vi "2-1.vi"() -> ()   [LabVIEW 2019, in "AoC2022.lvlib"]
uses:
  AoC2022.lvlib
panel:
  out "Player 1":i32
  out "Player 2":i32
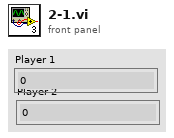
[diagram p1: front panel]
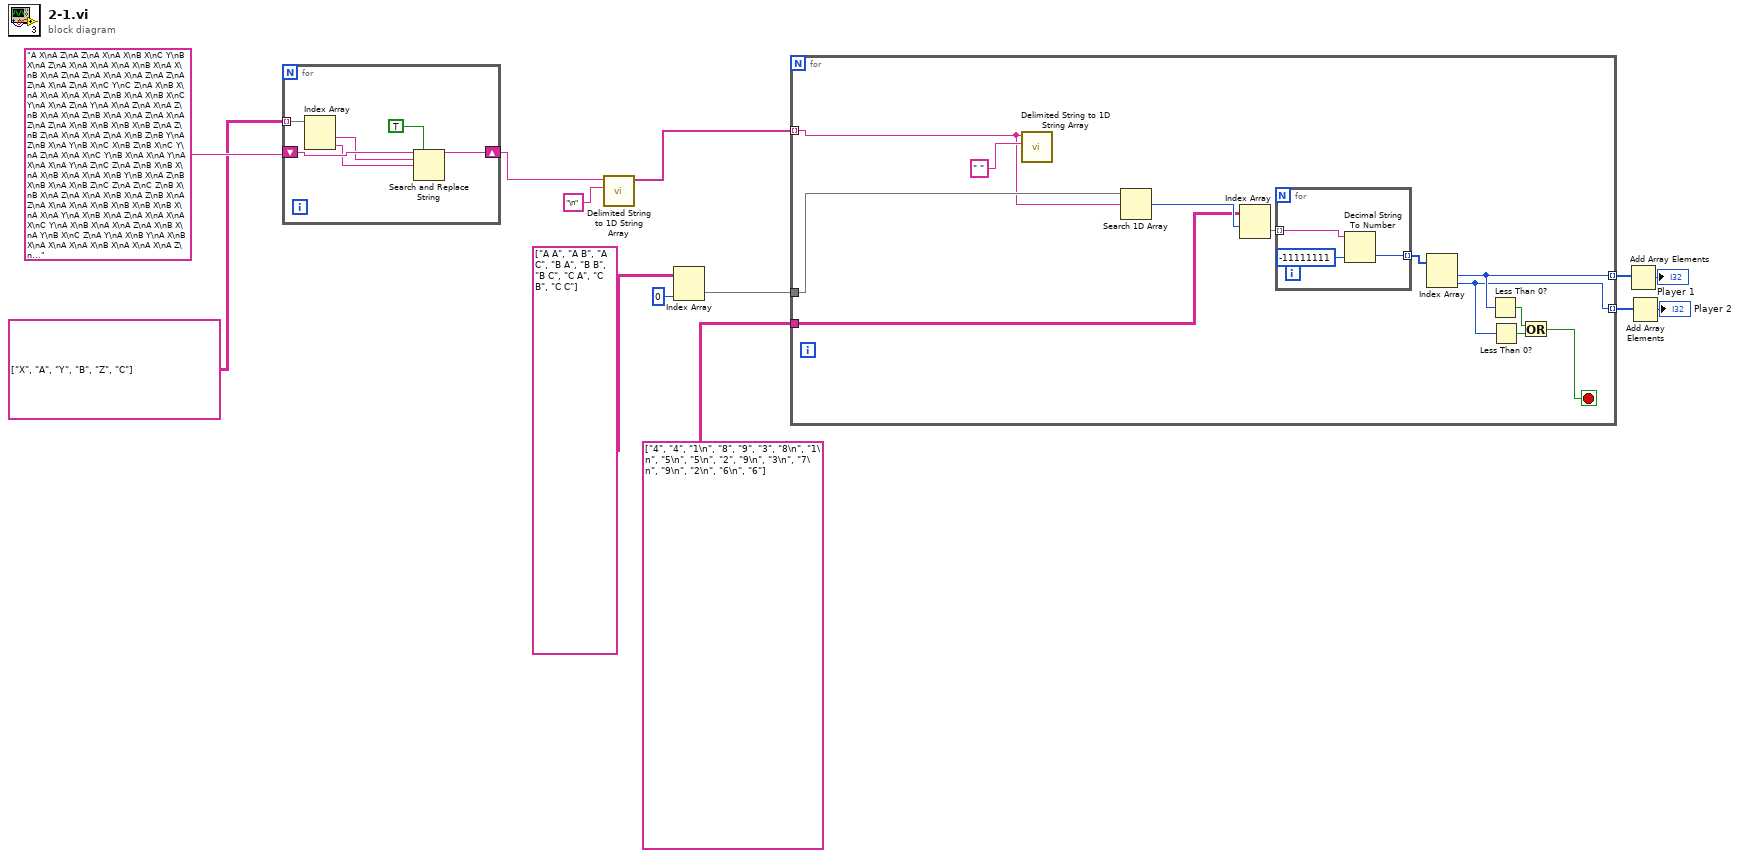
[diagram p0: block diagram]
diagram:
  n1 = for {
    tunnel: string[][] [["X", "A"], ["Y", "B"], ["Z", "C"]] -> [w18] mode=indexing
    shift-right: [w14] -> w1
    shift-left: "A X\nA Z\nA Z\nA X\nA X\nB X\nC Y\nB X\nA Z\nA X\nA X\nA X\nA X\nB X\nA X\nB X\nA Z\nA Z\nA X\nA X\nA Z\nA Z\nA Z\nA X\nA Z\nA X\nC Y\nC Z\nA X\nB X\nA X\nA X\nA X\nA Z\nB X\nA X\nB X\nC Y\nA X\nA Z\nA Y\nA X\nA Z\nA X\nA Z\nB X\nA X\nA Z\nB X\nA X\nA Z\nA X\nA Z\nA Z\nA X\nB X\nB X\nB X\nB Z\nA Z\nB Z\nA X\nA X\nA Z\nA X\nB Z\nB Y\nA Z\nB X\nA Y\nB X\nC X\nB Z\nB X\nC Y\nA Z\nA X\nA X\nC Y\nB X\nA X\nA Y\nA X\nA X\nA Y\nA Z\nC Z\nA Z\nB X\nB X\nA X\nB X\nA X\nA X\nB Y\nB X\nA Z\nB X\nB X\nA X\nB Z\nC Z\nA Z\nC Z\nB X\nB X\nA Z\nA X\nA X\nB X\nA Z\nB X\nA Z\nA X\nA X\nA X\nB X\nB X\nB X\nB X\nA X\nA Y\nA X\nB X\nA Z\nA X\nA X\nA X\nC Y\nA X\nB X\nA X\nA Z\nA X\nB X\nA Y\nB X\nC Z\nA Y\nA X\nB Y\nA X\nB X\nA X\nA X\nA X\nB X\nA X\nA X\nA Z\nA Z\nA X\nC Y\nB X\nB X\nA Z\nB X\nB Y\nC Y\nA X\nA X\nB Y\nA X\nB Y\nB X\nB X\nA X\nA Z\nB X\nB X\nA Y\nA X\nC Y\nC Y\nC Y\nA X\nB X\nA X\nA X\nA X\nB X\nB X\nC Y\nA X\nA Z\nA Z\nA X\nB X\nA Z\nA Z\nA X\nB X\nA X\nA Z\nA X\nC Z\nB X\nA X\nC Y\nC Y\nA Z\nB X\nB Z\nC Y\nB X\nA Y\nB Y\nA Z\nA X\nA X\nB X\nB Y\nA Z\nA X\nB X\nA X\nC X\nC Y\nA X\nB X\nA Z\nA X\nB X\nA X\nC Y\nC Y\nC Y\nA X\nA X\nA Z\nA X\nC Y\nA Z\nB Y\nA X\nC Y\nB Z\nB X\nB X\nA Z\nB X\nA Y\nC X\nA X\nB X\nA Z\nC Y\nA X\nA Z\nC Z\nA X\nC Y\nB X\nC Y\nC Z\nA Y\nA Z\nC Y\nA X\nA X\nA X\nA Y\nB X\nB X\nC Y\nC Y\nA X\nA Z\nC Y\nB Z\nB X\nC Z\nB X\nB X\nC Z\nA X\nA X\nB X\nB X\nA X\nA X\nB X\nB X\nB X\nC Y\nA X\nA X\nA X\nA X\nB X\nA X\nA X\nB X\nB Z\nA X\nB X\nA X\nC Y\nB Y\nA X\nB X\nA Y\nB Z\nB X\nA X\nB Z\nB X\nA Y\nA X\nB X\nA X\nA Z\nB X\nA X\nA X\nC Z\nA X\nB X\nA X\nB Y\nA Z\nA X\nB X\nA X\nA Z\nB X\nB X\nB Y\nB X\nA X\nC Y\nA X\nA X\nB X\nB Y\nA X\nA X\nA X\nC Z\nC Z\nB Y\nB X\nB Z\nA X\nA Y\nA X\nC Y\nB X\nA X\nA X\nA X\nA Z\nC Y\nA X\nA X\nC Y\nA X\nA X\nA X\nA Z\nA Y\nA X\nA Y\nC Z\nA Z\nA X\nB X\nA Z\nC Z\nC Y\nA Z\nA Z\nC Y\nC Z\nC Z\nA X\nB X\nB X\nB Z\nC Y\nA X\nA X\nA X\nA Z\nA X\nB X\nB X\nC X\nA X\nA X\nB X\nA Y\nA X\nA X\nB Y\nC Z\nA X\nA X\nA Y\nB X\nB X\nB X\nC Z\nA Z\nA Y\nB Y\nA X\nB X\nB X\nB X\nB Z\nA Y\nB Y\nA Z\nA Z\nC Z\nB X\nA X\nA Y\nA Y\nC Y\nB Y\nA X\nA X\nA X\nA X\nB Y\nA X\nA Y\nA X\nA Z\nB X\nB X\nA Y\nA X\nA Y\nA Y\nA Z\nB X\nB X\nA Z\nB X\nA X\nA Z\nA Z\nB X\nA Z\nA X\nA Y\nA Z\nA X\nA Z\nB Y\nA X\nC Y\nB X\nC X\nC Y\nB Z\nC Y\nC Y\nA X\nA X\nA Y\nB X\nC Z\nB X\nC Y\nA X\nA Z\nC Y\nA X\nA Z\nA Z\nB Y\nA X\nA X\nB X\nB Y\nA X\nA X\nB X\nA X\nB X\nA X\nB X\nA X\nB Y\nA Z\nB X\nB X\nB X\nB X\nA Y\nA X\nA Y\nA Y\nC Z\nB Z\nA X\nB Y\nA X\nC Z\nB X\nA X\nA X\nA X\nA X\nA X\nC Z\nC Z\nC Z\nA X\nC Y\nA X\nC X\nC Z\nA X\nB X\nA Z\nA Z\nA Z\nA X\nA Z\nA Z\nB Z\nA X\nB X\nA Z\nC Y\nA X\nA Z\nA Z\nA Z\nB Z\nB X\nA X\nB X\nB X\nB X\nB X\nB Y\nB X\nA X\nA X\nA Z\nA Z\nA Z\nB Y\nA X\nA X\nA Y\nB X\nB X\nA Z\nA X\nB X\nA X\nA X\nA Z\nC Y\nA X\nB X\nA X\nB X\nA X\nB X\nA Z\nB X\nA X\nA Z\nA Z\nB X\nA Y\nA X\nA Z\nC Y\nA X\nA X\nA X\nB Y\nB X\nA Y\nA Z\nC X\nB X\nC Y\nA X\nB X\nC Z\nC Z\nA X\nB X\nB X\nB Y\nB X\nB X\nA X\nA Z\nB Z\nB X\nA X\nB X\nB X\nB X\nA Z\nA X\nA X\nA Z\nB Y\nB Z\nA X\nA Z\nA Z\nA Z\nA X\nA X\nA X\nA X\nA X\nA X\nB X\nA Z\nB Z\nA X\nA Z\nC Y\nA Z\nA X\nA Y\nA Y\nB X\nB Y\nA Z\nA X\nB X\nB Y\nA X\nB X\nA X\nB X\nB X\nC Y\nA Z\nB X\nA X\nB X\nA X\nA Z\nA X\nA Z\nA X\nA X\nA X\nB X\nA Y\nA X\nA X\nB X\nC Z\nB X\nA X\nC Y\nA X\nB X\nA Z\nB Y\nB Z\nA X\nA X\nA X\nC Y\nA X\nA X\nA X\nB X\nC Z\nA Z\nA X\nC Z\nB X\nA Z\nA Y\nC Y\nC Y\nA Z\nB X\nC Z\nC Z\nA X\nA X\nA X\nA X\nA X\nB X\nC Y\nA Z\nA X\nB X\nA Z\nA X\nA Y\nA X\nB Z\nA X\nB X\nA X\nA X\nA X\nA Y\nB X\nC Y\nA X\nA Z\nC Y\nA Z\nA X\nA Y\nA X\nA Z\nA X\nA Y\nC Y\nA Y\nA Z\nA X\nA X\nA X\nA Z\nA X\nB X\nA Y\nA X\nB X\nA X\nA X\nB X\nA X\nB X\nC Z\nB X\nA Z\nA Z\nC Y\nB Y\nB X\nA Y\nB X\nB X\nA Y\nA X\nC X\nC Y\nB X\nA X\nC X\nC Z\nA X\nA Z\nB X\nB Z\nC Y\nA X\nC Y\nA Y\nB X\nB Y\nA X\nC Y\nA Z\nA X\nA X\nC Y\nC Y\nA X\nA Z\nB X\nA Y\nB X\nA Z\nA Z\nA Z\nA Z\nA X\nC Z\nB X\nB Y\nA X\nA Y\nA X\nB X\nC Y\nC Z\nB Z\nB X\nB Z\nA X\nA Z\nC Y\nA X\nB Y\nA X\nA Z\nA X\nC Z\nA X\nA Y\nB Y\nA X\nA X\nA X\nA Z\nB X\nB X\nB X\nA X\nC Y\nC X\nC Y\nC Z\nA X\nA X\nA Z\nA Z\nA X\nA X\nA X\nA X\nA X\nA X\nA X\nC Z\nA X\nB X\nA Z\nB X\nB X\nB X\nA Y\nA X\nA X\nB X\nA X\nB X\nA Z\nC Y\nB Y\nC Z\nB Y\nB X\nB X\nA X\nC Z\nA X\nB Y\nC Y\nB Y\nA Z\nA Y\nA X\nA X\nC Y\nB X\nB X\nA Z\nA X\nC Y\nC Y\nA Y\nA Z\nB X\nC Z\nA Z\nC Y\nA X\nA X\nA Z\nB X\nA X\nA X\nA Z\nB X\nC Z\nA X\nA X\nB X\nB Y\nA Z\nA X\nB X\nA X\nC Y\nB X\nB X\nB Z\nC Y\nA X\nB X\nA X\nA X\nA Y\nA Y\nA Z\nB X\nA Z\nB Y\nB X\nA X\nB Y\nA X\nA X\nA Z\nA X\nB X\nA Z\nA X\nA Z\nB X\nB X\nB X\nB Z\nC Y\nA Y\nA Y\nA Z\nA X\nB X\nB X\nA X\nA X\nB Y\nA X\nB X\nA Z\nB Z\nB X\nC Y\nA Z\nA X\nC Z\nA Y\nA Y\nB X\nA Y\nC Z\nA Z\nA X\nB X\nA Z\nC Y\nC X\nB X\nB Z\nA X\nA Y\nA X\nB X\nA X\nA X\nC Y\nB Z\nB Z\nB Y\nC Z\nC Y\nB X\nB Y\nC Y\nA Z\nB X\nA X\nA X\nA X\nA X\nA X\nA X\nB X\nB X\nB X\nA X\nC Y\nA X\nA Y\nA Z\nB Y\nC Y\nA Z\nA X\nA X\nA Z\nA Y\nB X\nA Y\nA X\nA X\nC Z\nA X\nA X\nB X\nA X\nA Z\nA Z\nA X\nA X\nA X\nB X\nA X\nA X\nA X\nA Z\nA X\nB X\nB Z\nC Y\nA X\nA Z\nB X\nB X\nB X\nA X\nB X\nA X\nB X\nA Y\nB Y\nC Y\nA X\nC Z\nB Z\nA Z\nA X\nA X\nA Z\nA Y\nA Z\nA X\nA X\nB X\nA X\nA X\nA Z\nC Z\nB X\nB Y\nA Z\nB X\nA Z\nA X\nA X\nA X\nC Y\nC Y\nA Z\nA X\nA X\nB Y\nA Y\nA X\nB Z\nB X\nB Z\nB X\nB Y\nB X\nA Y\nA Z\nC Y\nB X\nA X\nA X\nB X\nB Z\nA X\nC X\nA X\nA X\nA X\nA X\nA X\nA X\nB X\nA X\nC Z\nA Y\nB X\nB X\nB Z\nA X\nB X\nB Z\nB X\nA Z\nA X\nB X\nA X\nA Y\nB X\nA Z\nC Z\nB X\nC Z\nA X\nA X\nC Y\nA Z\nC Y\nA Z\nA X\nB X\nA X\nC Y\nA Z\nA X\nA X\nB X\nB X\nA Z\nB Y\nB X\nA X\nA Z\nA X\nB X\nA X\nA Z\nA Z\nA Y\nA Y\nA X\nC Z\nA Z\nA Z\nA X\nB X\nA Y\nB Z\nA X\nA Z\nA X\nC Z\nB X\nA Z\nC Z\nA X\nC X\nA Z\nA X\nA X\nB Z\nA X\nB X\nA X\nB X\nC Z\nA X\nB X\nA Z\nB X\nC Y\nB X\nA Z\nA X\nA Y\nC Z\nA Z\nB X\nA Z\nA Y\nA Z\nB X\nA X\nB X\nC Y\nB X\nA X\nC Y\nA X\nA X\nB Y\nA X\nB Y\nA X\nA X\nA X\nB X\nA X\nA X\nC Z\nA X\nB X\nA Y\nA Y\nB Z\nA Z\nA Y\nA X\nB X\nB Y\nA Z\nB Y\nA X\nA Z\nA X\nA Z\nB X\nA X\nA X\nB X\nA Y\nB X\nB X\nA X\nA Z\nB X\nA Y\nB X\nA Z\nB X\nB X\nB X\nB X\nA Y\nA Z\nB X\nB Y\nB X\nC Y\nC Y\nC Y\nB X\nB X\nA Y\nA X\nB X\nB X\nA X\nB X\nA X\nA Z\nA Z\nA Z\nB X\nA X\nA X\nA Y\nA X\nA X\nC Y\nB X\nC Y\nA X\nA Y\nC Z\nA X\nB X\nA Z\nA X\nA X\nA Z\nA X\nB Z\nA X\nA Z\nA X\nC Y\nA Y\nC X\nA X\nC Y\nB X\nB X\nA Z\nA X\nA X\nA X\nB X\nA X\nC Y\nC Y\nA Y\nA X\nC Z\nA X\nB X\nB Y\nA Z\nA X\nB X\nB X\nA X\nA Z\nC Y\nB X\nA Y\nA X\nA Z\nB X\nA X\nA Z\nB X\nA Y\nB Z\nA Z\nC Z\nC Y\nA Z\nA X\nA X\nA Z\nB X\nA X\nB X\nA X\nA X\nB X\nA Z\nA X\nC Z\nB X\nA Z\nB Y\nA Z\nA X\nA Z\nB X\nA X\nA X\nA Y\nB X\nC Z\nB X\nA X\nA X\nA Z\nB X\nC X\nB X\nB X\nA Z\nB Y\nB X\nA Z\nC Y\nA X\nA X\nB X\nB X\nA X\nB X\nA Z\nA X\nA X\nA Z\nA X\nA X\nB X\nB X\nA X\nA Z\nA Y\nA X\nA X\nC Y\nB X\nA X\nB X\nC Z\nA Z\nB X\nA X\nA X\nA X\nC Y\nA X\nA X\nA X\nA Z\nB Y\nB X\nA X\nA X\nA Z\nB X\nC Z\nB X\nA Z\nA Z\nA X\nA Y\nB Y\nB X\nA Z\nA Z\nA X\nA Y\nB X\nA X\nA Z\nB X\nA Y\nA Z\nA Z\nB X\nC Z\nA X\nA X\nB X\nB X\nA X\nA Y\nA Y\nC Z\nB X\nA X\nA Z\nC Y\nB X\nA Z\nA X\nB X\nB Y\nA X\nB X\nA Y\nB X\nA X\nA Z\nB X\nB X\nC Y\nB X\nB X\nB Y\nA X\nA X\nB X\nB X\nA X\nB X\nC Y\nA X\nA X\nA Z\nA Z\nB X\nA Y\nB X\nB Y\nA X\nA Z\nA X\nA Z\nA X\nB Y\nB X\nB X\nA X\nB X\nA X\nB X\nB X\nA X\nB X\nC X\nA Z\nA Z\nA X\nA X\nA Z\nA X\nB X\nA X\nA X\nA Z\nA Z\nA X\nA X\nB X\nC Y\nA Z\nA X\nA X\nA Y\nA X\nB Z\nC Z\nA Z\nB X\nA X\nB X\nA X\nB X\nB X\nA Y\nB Y\nA X\nB X\nB Y\nC Y\nB Z\nB Y\nB Y\nA Z\nA X\nA Y\nA X\nA Z\nA Z\nA X\nA X\nA X\nA X\nA Y\nC Y\nA X\nA Y\nA Z\nA Z\nB X\nA X\nA X\nA Z\nB Y\nB X\nB X\nA X\nB Z\nB Z\nA Y\nB X\nA Y\nA X\nB X\nC Z\nA X\nA Y\nB X\nA X\nB Z\nC Y\nA Z\nA X\nA Z\nA X\nA X\nA X\nA X\nC Y\nB X\nA X\nA X\nC Y\nC Y\nA Z\nC Y\nA Z\nA Y\nC X\nB X\nC Y\nA Z\nA X\nB X\nB Z\nB X\nB X\nB X\nB X\nB X\nA X\nA Z\nB X\nA Y\nA X\nA Y\nB X\nA X\nA X\nA X\nB Z\nB Z\nB X\nB X\nA Y\nA X\nB Y\nB X\nB Y\nC Y\nA X\nA X\nC Y\nA X\nB X\nB X\nB X\nC Z\nB X\nA Z\nB X\nB X\nA X\nB Z\nA Z\nA Z\nA X\nA Z\nA Y\nA Z\nB X\nA X\nB X\nA X\nA X\nA X\nB X\nA X\nB X\nA X\nA X\nB X\nA Z\nA X\nA Z\nC Y\nA X\nB X\nA X\nA X\nB X\nB X\nC Z\nA X\nA X\nB X\nA X\nA Y\nA X\nA X\nA Z\nA X\nA X\nB X\nA X\nA X\nA X\nA Y\nC Z\nA Z\nA Z\nA X\nB X\nA Z\nA X\nA X\nA X\nC Y\nC Y\nA Z\nC Y\nB X\nA X\nB X\nB X\nA Z\nA Z\nA Y\nB X\nA Z\nA X\nA Z\nA X\nA X\nA X\nA Z\nA Z\nB X\nA X\nA X\nB X\nB X\nA Z\nB X\nA X\nA X\nB X\nB X\nB X\nA X\nA X\nA Z\nA X\nA X\nB Y\nB Y\nC Y\nA Y\nA Y\nB X\nB X\nC Y\nA X\nB X\nA X\nA X\nA Z\nA Y\nA X\nB X\nA X\nB X\nA X\nA Z\nA X\nC Y\nB X\nB X\nA X\nB X\nA X\nA X\nA Z\nC Y\nB X\nB X\nA X\nA X\nA Z\nA Z\nB Y\nA X\nB X\nA Y\nC Z\nB X\nA X\nA Z\nB Y\nA Z\nB X\nB X\nB X\nA X\nA Z\nA Z\nB Y\nA Y\nB X\nB Y\nA Y\nA Z\nA X\nA X\nB X\nB X\nA Y\nB X\nA X\nA X\nC Y\nB X\nA X\nC X\nC Z\nA X\nA X\nC Y\nC Z\nA Z\nA X\nC Y\nC Y\nC Y\nA X\nA Y\nA Z\nA X\nC Z\nA X\nC X\nB X\nB Y\nB Z\nA X\nA X\nA X\nA Z\nB X\nB X\nC X\nA X\nC Z\nC Y\nA X\nA X\nB X\nB X\nA X\nA X\nA X\nA Z\nA Z\nB X\nA Z\nB Y\nA Y\nA Y\nA Z\nB X\nA Y\nA X\nA X\nB X\nA Z\nB X\nA Y\nA X\nB X\nA X\nB X\nA X\nB X\nB Z\nA Z\nA Y\nA Z\nA X\nB X\nB X\nC Y\nB X\nA X\nB X\nA Y\nB X\nB X\nC Y\nB X\nA Z\nA Z\nC Y\nA X\nB X\nB X\nA X\nB X\nA Z\nA X\nA X\nA Z\nA Z\nC Z\nA X\nA X\nA X\nA X\nA X\nA X\nA Z\nC Y\nA X\nC Y\nA X\nB X\nC Y\nB X\nA Y\nB X\nB X\nB X\nA X\nA X\nA X\nC Y\nA Z\nA Z\nB X\nA X\nA Z\nB X\nB X\nA X\nA X\nB Z\nA X\nB Z\nB X\nA X\nA X\nA X\nB X\nA X\nC Y\nA Y\nA X\nA X\nB X\nA Y\nA X\nC Y\nC Y\nB X\nB X\nA X\nA X\nC Y\nB Y\nC Y\nA X\nB X\nA Y\nB Z\nB X\nB X\nA Y\nB X\nA Z\nC Y\nB X\nB X\nB Y\nA X\nA X\nA X\nC Y\nB X\nA Y\nB X\nA Z\nB Y\nA X\nA X\nA X\nA X\nA X\nA X\nB X\nC Z\nB X\nB X\nA X\nA X\nC Y\nA X\nA X\nA X\nA X\nB Z\nB X\nA Z\nB Z\nC Z\nC Y\nB X\nB X\nC Z\nA Z\nA Y\nA Z\nA Y\nC Z\nA X\nA X\nA Z\nA X\nA Z\nA X\nB Z\nB X\nB X\nC Z\nB X\nC Y\nC Y\nB X\nA X\nA X\nA X\nB Y\nA X\nC Y\nB Y\nC Y\nB Y\nA Z\nB X\nA X\nA Z\nB X\nB Z\nA Z\nA X\nA X\nA Y\nA X\nA X\nA Z\nB X\nB X\nB X\nB X\nB X\nA X\nA X\nA X\nA Z\nA Z\nA Y\nA X\nA Z\nA Z\nB X\nA X\nB X\nB X\nA Z\nB Y\nA X\nA X\nA X\nA X\nB X\nA Y\nA X\nC X\nA Z\nA X\nC Z\nC Y\nB X\nA Z\nA Z\nB X\nC Y\nA X\nA Z\nA X\nB Y\nC Y\nA X\nA X\nA Z\nA X\nC Y\nA Z\nA X\nA X\nA X\nC Y\nB X\nA X\nB Y\nA Z\nA X\nA Z\nB X\nA Z\nA Z\nA X\nA X\nC Z\nB X\nA Z\nA X\nB Z\nA Z\nA Z\nB X\nA X\nA Z\nA Y\nA X\nA Z\nA Z\nC X\nC Z\nB X\nB X\nA Z\nA X\nB X\nA X\nA X\nA X\nA Z\nB X\nA Z\nA X\nB X\nA X\nA X\nC Z\nB X\nC Y\nA X\nB X\nA Z\nA Z\nA X\nB Z\nB X\nA Z\nA Z\nA X\nC Y\nA X\nB X\nC Y\nB X\nB X\nA Z\nB X\nA Z\nC Y\nB X\nA Y\nB X\nA Z\nB Z\nA Z\nB X\nA X\nB Z\nA X\nA Y\nB Z\nC Y\nC Y\nB X\nA X\nA X\nA X\nA X\nB Z\nA X\nA X\nA X\nC Y\nC X\nB Y\nB X\nB X\nB X\nA Y\nA X\nA Z\nA X\nB X\nA Z\nC Y\nA X\nA Z\nA Z\nA X\nA X\nA X\nA X\nA Z\nA X\nA X\nB X\nC Z\nB X\nC Z\nB Y\nB X\nA Z\nA Z\nA Z\nB Y\nA Y\nA Z\nB X\nC Y\nA X\nB X\nA Z\nC Y\nA Y\nB X\nA X\nA Y\nA X\nA Z\nB X\nA Z\nB Y\nB X\nA X\nB X\nA X\nA X\nA X\nA Y\nB X\nA Y\nA X\nB X\nA X\nA X\nC Y\nA X\nA X\nB Z\nA Z\nA Z\nA X\nC Y\nB X\nB X\nC Y\nA Z\nC Y\nA X\nA X\nB X\nB X\nA X\nA Z\nB Y\nB X\nA Z\nB X\nA X\nB X\nA Z\nC Y\nA X\nB X\nA X\nA X\nA Z\nA X\nB X\nC Z\nA X\nA X\nA Y\nB X\nA Z\nB X\nB X\nB Y\nA X\nA Z\nA X\nA Z\nB X\nB X\nA X\nA X\nB Z\nA X\nC Y\nB X\nA X\nA Z\nA Z\nB X\nC Y\nC Y\nB Y\nA Z\nC Z\nA X\nB X\nA X\nA X\nB Y\nB X\nA X\nA X\nA Y\nA Z\nB X\nA X\nA X\nA Z\nA X\nA X\nB X\nB X\nA Y\nA X\nB X\nA Z\nB Z\nB X\nA Z\nA X\nA Z\nB X\nC Y\nA X\nA X\nB X\nA Z\nB X\nA Z\nC Z\nA Z\nA X\nC Y\nA X\nB X\nB Z\nA X\nB X\nC X\nA X\nB Y\nA X\nA X\nC Y\nA X\nB Y\nA X\nA X\nA X\nB X\nA X\nB X\nA Z\nC Y\nA X\nC Z\nA X\nB X\nA Z\nA X\nC Z\nC Z\nA X\nA Y\nA Z\nA X\nB X\nB X\nA Z\nB X\nA X\nB X\nB Y\nB X\nB X\nC Z\nA Y\nA X\nA Z\nB Z\nA X\nA Z\nA Z\nA Y\nB X\nA Y\nA X\nA X\nB X\nA Z\nB Z\nA X\nA Z\nA Z\nA Z\nC Y\nA X\nB Z\nB X\nA Z\nB X\nA Z\nA Y\nA X\nC Z\nC X\nA Y\nA X\nA Z\nA X\nA X\nA Z\nA Y\nA Z\nA Y\nA X\nC Y\nB X\nA Z\nA X\nA X\nC Y\nA X\nA X\nB Z\nA Z\nC Y\nA X\nA X\nA X\nB X\nC Y\nA X\nA Y\nB X\nA X\nA X\nB Y\nA Z\nA X\nA X\nB X\nA Z\nA Y\nC Y\nC Z\nC Y\nA X\nC Y\nC Y\nA X\nA Y\nC Y\nB X\nA X\nB X\nA X\nA X\nB X\nA X\nA Z\nC Y\nC Y\nB X\nA X\nB X\nC Z\nC Y\nB X\nA X\nA X\nA Y\nA X\nA Y\nA Z\nB X\nA Z\nA Z\nA X\nA X\nB X\nC Y\nB X\nA Z\nA X\nA X\nA X\nB X\nB Z\nB X\nB X\nB X\nA Z\nA X\nB Z\nA X\nB Z\nA X\nB Y\nC Z\nB Y\nC Z\nB Y\nB X\nA X\nA X\nC Y\nB X\nB X\nA X\nB Z\nA Z\nA Z\nA X\nA X\nA X\nB X\nB X\nB X\nC Y\nA X\nB X\nB X\nB Z\nB X\nA Z\nC Y\nA X\nC Z\nA Z" -> [w19]
    n2 = Index Array(array=w18) -> (element #1=w17:string, element #2=w16:string)  [unwired: 2 in]
    n3 = Search and Replace String(replace all?=TRUE ("replace all? (F)"), input string=w19, search string=w17, replace string=w16) -> (result string=w14:string)  [unwired: 4 in, 3 out]
  }
  n4 = call <vilib>:"Delimited String to 1D String Array.vi"("delimiter"="\n", "delimited string"=w1) -> ("string array"=w12:string[])  [unwired: 9 in]
  n5 = Index Array(array=string[][] [["A A"], ["A B"], ["A C"], ["B A"], ["B B"], ["B C"], ["C A"], ["C B"], ["C C"]], index (col)=0 ("disabled index (col)")) -> (element=w9:string[])  [unwired: 1 in]
  n6 = for {
    tunnel: w12 -> [w29] mode=indexing
    tunnel: w9 -> [w30]
    tunnel: [w23] -> w8 mode=indexing
    tunnel: string[][] [["4", "4"], ["1\n", "8"], ["9", "3"], ["8\n", "1\n"], ["5\n", "5\n"], ["2", "9\n"], ["3\n", "7\n"], ["9\n", "2\n"], ["6\n", "6"]] -> [w27]
    tunnel: [w24] -> w4 mode=indexing
    stop <- w20 stop-if-true
    n7 = call <vilib>:"Delimited String to 1D String Array.vi"("delimiter"=" ", "delimited string"=w29) -> ()  [unwired: 9 in, 1 out]
    n8 = Search 1D Array(1D array=w30, element=w29) -> (index of element=w28:i32)  [unwired: 1 in]
    n9 = Index Array(array=w27, index (row)=w28) -> (element=w26:string[])  [unwired: 1 in]
    n10 = for {
      tunnel: [w34] -> w25 mode=indexing
      tunnel: w26 -> [w32] mode=indexing
      n11 = Decimal String To Number(string=w32, default (0L)=-11111111 ("default (0 I32)")) -> (number=w34:i32)  [unwired: 1 in, 1 out]
    }
    n12 = Index Array(array=w25) -> (element #1=w24:i32, element #2=w23:i32)  [unwired: 2 in]
    n13 = Less Than 0?(x=w24) -> (x < 0?=w21:bool)
    n14 = Less Than 0?(x=w23) -> (x < 0?=w22:bool)
    n15 = Or(x=w21, y=w22) -> (x .or. y?=w20:bool)
  }
  n16 = Add Array Elements(numeric array=w4) -> (sum=→"Player 1":i32)
  n17 = Add Array Elements(numeric array=w8) -> (sum=→"Player 2":i32)
